vi "Fetch Multi Eval Meas List Segment Modulation Extreme Results.vi"(8 "error in (no error)":errorcluster, 9 "Segment (1)":T2=1, 10 "Instance (1)":T3=1, 11 "VISA resource name":refnum<visa-resource-name>) -> (0 "error out":errorcluster, 1 "Results":dbl[](array[numeric]) format="%^.3e", 2 "Reliability":T1, 3 "VISA resource name out":refnum<visa-resource-name>, 4 "Expired Statistics":i32, 5 "Out Of Tolerance":i32)   [LabVIEW 2020, in "Rohde&Schwarz CMWXP NR FR1 Measurement.lvlib"]
doc: "Returns extreme modulation single value results for segment <no> in list mode.\n\nAttribute:\nRSCMWXPNRFR1M_ATTR_FETCH_MULTI_EVAL_MEAS_LIST_SEGMENT_MODULATION_EXTREME_RESULTS\n\nRemote-control command:\nFETCh:NRSub:MEAS<i>:MEValuation:LIST:SEGMent<no>:MODulation:EXTReme?"
uses:
  <instrlib>/Rohde&Schwarz CMWXP NR FR1 Measurement/Rohde&Schwarz CMWXP NR FR1 Measurement.lvlib
  <instrlib>/Rohde&Schwarz CMWXP NR FR1 Measurement/Private/_Instance.ctl
  <instrlib>/Rohde&Schwarz CMWXP NR FR1 Measurement/Private/_Segment.ctl
  <instrlib>/Rohde&Schwarz CMWXP NR FR1 Measurement/Private/_SegReliability.ctl
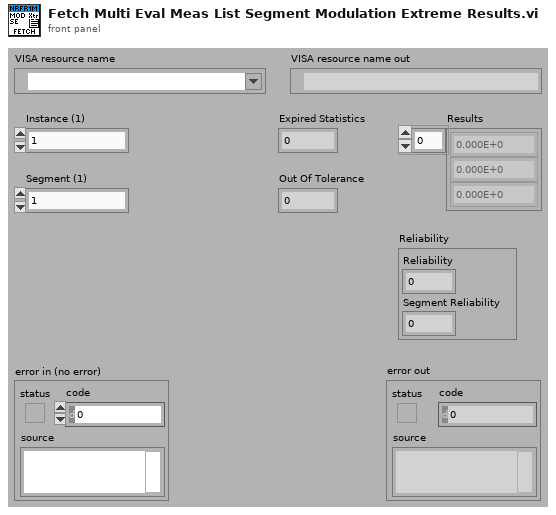
[diagram p1: front panel]
types:
  T1 = typedef "Rohde&Schwarz CMWXP NR FR1 Measurement.lvlib/_SegReliability.ctl" = cluster{"Reliability":i32, "Segment Reliability":i32}
  T2 = typedef "Rohde&Schwarz CMWXP NR FR1 Measurement.lvlib/_Segment.ctl" = i32
  T3 = typedef "Rohde&Schwarz CMWXP NR FR1 Measurement.lvlib/_Instance.ctl" = i32
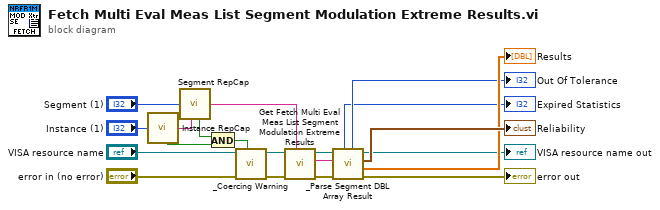
[diagram p0: block diagram]
diagram:
  n1 = call <instrlib>:"Instance RepCap.vi"("Instance In"="Instance (1)") -> ("In Range?"=w15:bool, "RepCap Identifier Out"=w14:string)  [unwired: 1 in]
  n2 = call <instrlib>:"Segment RepCap.vi"("Segment In"="Segment (1)", "RepCap String In (\"\")"=w14) -> ("In Range?"=w13:bool, "RepCap Identifier Out"=w12:string)
  n3 = And(x=w13, y=w15) -> (x .and. y?=w16:bool)
  n4 = call <instrlib>:"_Coercing Warning.vi"("In Range?"=w16, "error in (no error)"="error in (no error)", "VISA resource name"="VISA resource name") -> ("error out"=w10:errorcluster, "VISA resource name out"=w11:refnum<visa-resource-name>)  [unwired: 7 in]
  n5 = call "Get Fetch Multi Eval Meas List Segment Modulation Extreme Results"("Repeated Capabilities"=w12, "error in (no error)"=w10, "instrument handle"=w11) -> ("error out"=w7:errorcluster, "Fetch Multi Eval Meas List Segment Modulation Extreme Results"=w8:string, "instrument handle out"=w9:refnum<visa-resource-name>)  [unwired: 6 in]
  n6 = call <instrlib>:"_Parse Segment DBL Array Result.vi"("error in (no error)"=w7, "Input String"=w8, "VISA resource name"=w9) -> ("error out"=→"error out":errorcluster, "Results"=→"Results":dbl[], "Reliability Results"=→"Reliability":T1, "VISA resource name out"=→"VISA resource name out":refnum<visa-resource-name>, "Out Of Tolerance"=→"Out Of Tolerance":i32, "Statistic Expired"=→"Expired Statistics":i32)  [unwired: 3 in]
